vi "XML - Set Rx Channels.vi"(8 "error in (no error)":errorcluster, 9 "Rx Channel Paths":string[](array[string]), 10 "Rx Channel Names":string[](array[string]), 11 "Item Ref in":T1 format="%.0x") -> (0 "error out":errorcluster, 3 "Item Ref out":T1=18446744073709551615 format="%.0x")   [LabVIEW 2019]
uses:
  <vilib>/NI VeriStand/Custom Device API/Custom Device Item Ref.ctl
  Shared/Constants.vi
  <vilib>/NI VeriStand/Custom Device API/Get Item Property (Dependent Node Pointer).vi
  <vilib>/NI VeriStand/Custom Device Tools/Custom Device Utility Library/Custom Device Utility Library.lvlib
  <vilib>/NI VeriStand/Custom Device API/Custom Device API.lvlib
  UDP-Custom-Device System Explorer.lvlib
  Shared/UDP-Custom-Device Shared.lvlib
  Property Accessors/Shared Packet Accessors.lvlib
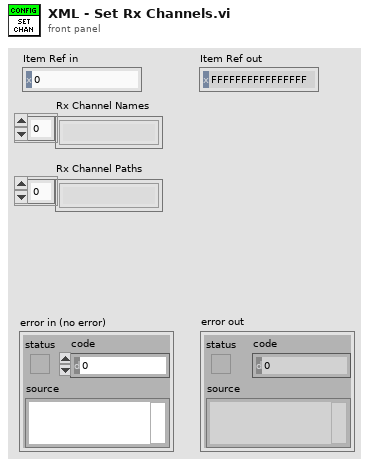
[diagram p1: front panel]
types:
  T1 = typedef "Custom Device API.lvlib/Custom Device Item Ref.ctl" = u64
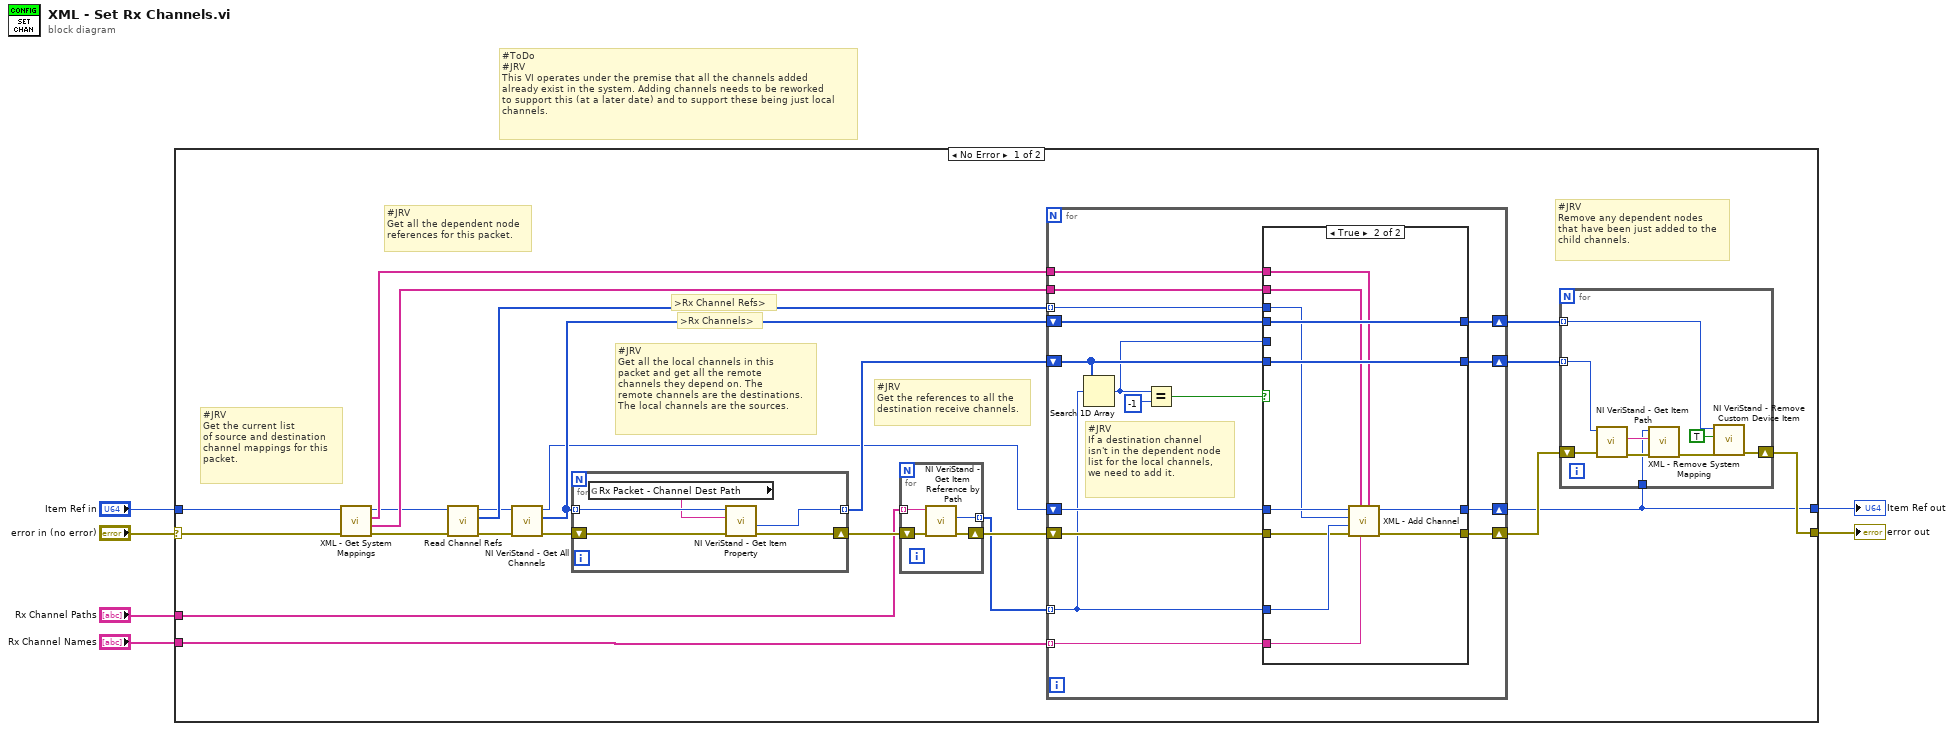
[diagram p0: block diagram]
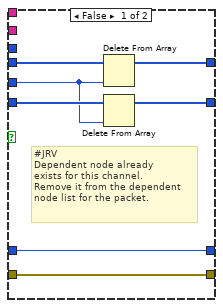
[diagram p2: hidden frame]
diagram:
  # "#ToDo\n#JRV\nThis VI operates under the premise that all the channels added\nalready exist in the system. Adding channels needs to be reworked\nto support this (at a later date) and to support these being just local\nchannels."
  n1 = case shown="No Error" "error in (no error)" {
    selector: "error in (no error)" -> [w18 w82]
    tunnel: "Item Ref in" -> [w17 w83]
    tunnel: [w16 w83] -> w4
    tunnel: [w26 w82] -> w3
    tunnel: "Rx Channel Paths" -> [w13 _]
    tunnel: "Rx Channel Names" -> [w12 _]
    frame No Error {
      # "#JRV\nRemove any dependent nodes\nthat have been just added to the\nchild channels."
      # "#JRV\nGet the references to all the\ndestination receive channels."
      # "#JRV\nGet all the local channels in this\npacket and get all the remote \nchannels they depend on. The\nremote channels are the destinations.\nThe local channels are the sources."
      # "#JRV\nGet all the dependent node\nreferences for this packet."
      # "#JRV\nGet the current list\nof source and destination\nchannel mappings for this\npacket."
      # ">Rx Channels>"
      # ">Rx Channel Refs>"
      n2 = call "XML - Get System Mappings.vi"("error in (no error)"=w18, "Item Ref in"=w17) -> ("error out"=w7:errorcluster, "Channel Path Destinations"=w19:string[], "Channel Path Sources"=w20:string[], "Item Ref out"=w8:T1)  [unwired: 6 in]
      n3 = call "Read Channel Refs.vi"("error in (no error)"=w7, "Node Ptr"=w8) -> ("error out"=w9:errorcluster, "Dependent Node Refs"=w11:T1[], "Node Ptr out"=w10:T1)  [unwired: 7 in]
      n4 = call <vilib>:"NI VeriStand - Get All Channels.vi"("error in"=w9, "Section Ref in"=w10) -> ("error out"=w29:errorcluster, "Channel Refs"=w28:T1[], "Section Ref out"=w15:T1)  [unwired: 6 in, 1 out]
      n5 = for {
        tunnel: w28 -> [w81] mode=indexing
        tunnel: [w79] -> w24 mode=indexing
        shift-right: [w78] -> w23
        shift-left: w29 -> [w80]
        n6 = global read "Constants.vi" "Rx Packet - Channel Dest Path"() -> (w77:string)
        n7 = call-poly <vilib>:"NI VeriStand - Get Item Property.vi"("error in (no error)"=w80, "Property Name"=w77, "Item Ref in"=w81) -> ("error out"=w78:errorcluster, "Dependent Node Ref"=w79:T1)  [unwired: 5 in, 2 out]
      }
      n8 = for {
        tunnel: w13 -> [w76] mode=indexing
        tunnel: [w75] -> w14 mode=indexing
        shift-right: [w73] -> w22
        shift-left: w23 -> [w74]
        n9 = call <vilib>:"NI VeriStand - Get Item Reference by Path.vi"("error in (no error)"=w74, "Item Path in"=w76) -> ("error out"=w73:errorcluster, "Item Ref"=w75:T1)  [unwired: 6 in, 2 out]
      }
      n10 = for {
        tunnel: w14 -> [w40] mode=indexing
        shift-right: [w39] -> w27
        shift-left: w22 -> [w43]
        tunnel: w12 -> [w41] mode=indexing
        tunnel: w11 -> [w38] mode=indexing
        shift-right: [w35] -> w25
        shift-left: w28 -> [w36]
        shift-right: [w33] -> w21
        shift-left: w24 -> [w34]
        tunnel: w20 -> [w30]
        tunnel: w19 -> [w31]
        shift-right: [w37] -> w16
        shift-left: w15 -> [w42]
        # "#JRV\nIf a destination channel\nisn't in the dependent node\nlist for the local channels,\nwe need to add it."
        n11 = Search 1D Array(1D array=w34, element=w40) -> (index of element=w32:i32)  [unwired: 1 in]
        n12 = Equal?(x=w32, y=-1) -> (x = y?=w44:bool)
        n13 = case shown="True" w44 {
          tunnel: w43 -> [w47 w58]
          tunnel: w42 -> [w46 w55]
          tunnel: w41 -> [_ w56]
          tunnel: w40 -> [_ w59]
          tunnel: [w47 w57] -> w39
          tunnel: w38 -> [_ w53]
          tunnel: [w46 w54] -> w37
          tunnel: w36 -> [w52 w63]
          tunnel: [w51 w63] -> w35
          tunnel: w32 -> [w48 _]
          tunnel: w34 -> [w50 w62]
          tunnel: [w49 w62] -> w33
          tunnel: w31 -> [_ w61]
          tunnel: w30 -> [_ w60]
          frame False {
            # "#JRV\nDependent node already\nexists for this channel.\nRemove it from the dependent\nnode list for the packet."
            n14 = Delete From Array(array=w52, index=w48) -> (array with subset deleted=w51:T1[])  [unwired: 1 in, 1 out]
            n15 = Delete From Array(array=w50, index=w48) -> (array with subset deleted=w49:T1[])  [unwired: 1 in, 1 out]
          }
          frame True {
            n16 = call "XML - Add Channel.vi"("Channel Path Sources"=w60, "Rx Channel Name"=w56, "Channel Path Destinations"=w61, "error in (no error)"=w58, "Rx Channel Ref"=w59, "Dependent Node Ref"=w53, "Rx Section Ref in"=w55) -> ("error out"=w57:errorcluster, "Rx Section Ref in"=w54:T1)  [unwired: 3 in]
          }
        }
      }
      n17 = for {
        shift-right: [w72] -> w26
        shift-left: w27 -> [w70]
        tunnel: w25 -> [w65] mode=indexing
        tunnel: w21 -> [w66] mode=indexing
        tunnel: w16 -> [w64]
        n18 = call <vilib>:"NI VeriStand - Get Item Path.vi"("error in (no error)"=w70, "Item Ref in"=w66) -> ("error out"=w69:errorcluster, "Path"=w67:string)  [unwired: 6 in, 2 out]
        n19 = call "XML - Remove System Mapping.vi"("error in (no error)"=w69, "Channel Path Destination"=w67, "Item Ref in"=w64) -> ("error out"=w68:errorcluster)  [unwired: 7 in, 1 out]
        n20 = call <vilib>:"NI VeriStand - Remove Custom Device Item.vi"("error in (no error)"=w68, "Force Delete (F)"=TRUE, "Item Ref in"=w65) -> ("error out"=w72:errorcluster)  [unwired: 7 in, 1 out]
      }
    }
    frame Error {
    }
  }
  "Item Ref out" <- w4
  "error out" <- w3
